vi "YKMW100 Receive String-clear buff.vi"(0 "VISA session":refnum<visa-resource-name>="MW100", 2 "Semiphore":T1, 9 "Timeout (25000)":u32=100, 11 "error in (no error)":errorcluster, 13 "Source (\"\")":string) -> (4 "dup VISA session":refnum<visa-resource-name>, 8 "Read Buffer":string, 15 "error out":errorcluster)   [LabVIEW 2009]
doc: "This VI receives ASCII code string which ends with terminator \"CRLF\" from the instrument. \nThis VI returns read buffer except CRLF."
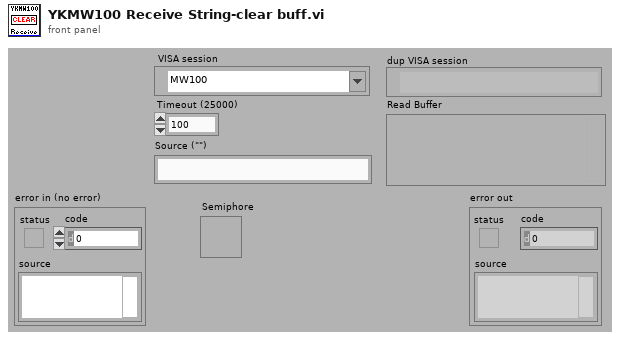
[diagram p1: front panel]
types:
  T1 = typedef "Semaphore RefNum" = refnum<k1>
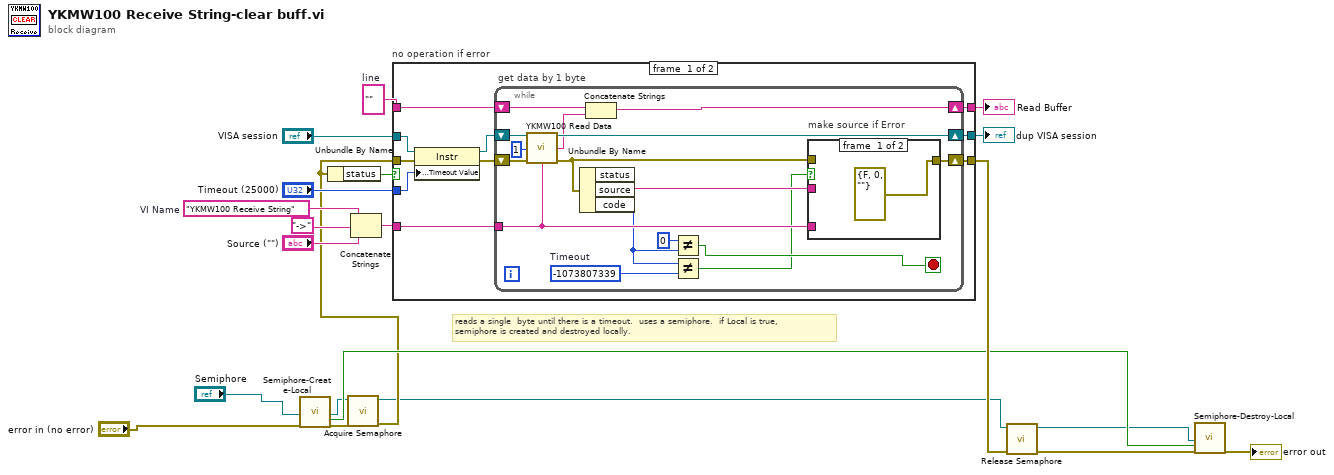
[diagram p0: block diagram]
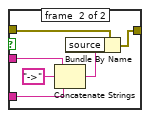
[diagram p2: hidden frame]
diagram:
  w14 = "YKMW100 Receive String"  # VI Name
  w17 = ""  # line
  # "reads a single  byte until there is a timeout.  uses a semiphore.  if Local is true, \nsemiphore is created and destroyed locally."
  n1 = call "Semiphore-Create-Local.vi"("Semiphore"="Semiphore", "error in (no error)"="error in (no error)") -> ("semaphore"=w4:T1, "Local?"=w7:bool, "error out"=w6:errorcluster)  [unwired: 15 in]
  n2 = call <vilib>:"Acquire Semaphore.vi"("error in (no error)"=w6, "semaphore"=w4) -> ("error out"=w5:errorcluster, "semaphore out"=w1:T1)  [unwired: 3 in, 1 out]
  n3 = Unbundle By Name(w5) -> ("status"=w20:bool)
  n4 = Concatenate Strings(w14, "->", "Source (\"\")") -> (w12:string)
  n5 = case "no operation if error" shown="False" w20 {
    tunnel: "VISA session" -> [w24 w57]
    tunnel: [w31 w57] -> w18
    tunnel: [w27 w56] -> w9
    tunnel: w5 -> [w26 w56]
    tunnel: w12 -> [w29 _]
    tunnel: [w28 w55] -> w19
    tunnel: w17 -> [w30 w55]
    tunnel: "Timeout (25000)" -> [w22 _]
    frame #0 {
      n6 = property class="Instr"(reference=w24, error in=w26, "General Settings:Timeout Value"=w22) -> (reference out=w23:refnum<visa-resource-name>, error out=w25:errorcluster)
      n7 = while "get data by 1 byte" {
        shift-left: w25 -> [w43]
        shift-right: [w45] -> w27
        tunnel: w29 -> [w39]
        shift-left: w30 -> [w47]
        shift-right: [w37] -> w28
        shift-right: [w42] -> w31
        shift-left: w23 -> [w44]
        stop <- w33 stop-if-true
        w36 = -1073807339  # Timeout
        n8 = call "YKMW100 Read Data.vi"("VISA session"=w44, "Byte (0)"=1, "error in (no error)"=w43, "Source (\"\")"=w39) -> ("dup VISA session"=w42:refnum<visa-resource-name>, "Read Buffer"=w38:string, "error out"=w41:errorcluster)  [unwired: 9 in]
        n9 = Unbundle By Name(w41) -> ("source"=w46:string, "code"=w35:i32)  [unwired: 1 out]
        n10 = Concatenate Strings(w47, w38) -> (w37:string)
        n11 = Not Equal?(x=0, y=w35) -> (x != y?=w33:bool)
        n12 = Not Equal?(x=w35, y=w36) -> (x != y?=w32:bool)
        n13 = case "make source if Error" shown="True" w32 {
          tunnel: w41 -> [_ w54]
          tunnel: [errorcluster {"status"=FALSE, "code"=0, "source"=""} ("error out") w53] -> w45
          tunnel: w46 -> [_ w51]
          tunnel: w39 -> [_ w49]
          frame #0 {
          }
          frame #1 {
            n14 = Concatenate Strings(w51, "->", w49) -> (w50:string)
            n15 = Bundle By Name(cluster=w54, "source"=w50) -> (w53:errorcluster)
          }
        }
      }
    }
    frame #1 {
    }
  }
  "dup VISA session" <- w18
  "Read Buffer" <- w19
  n16 = call <vilib>:"Release Semaphore.vi"("error in (no error)"=w9, "semaphore"=w1) -> ("error out"=w3:errorcluster, "semaphore out"=w2:T1)  [unwired: 4 in]
  n17 = call "Semiphore-Destroy-Local.vi"("Semiphore"=w2, "Local?"=w7, "error in (no error)"=w3) -> ("error out"=→"error out":errorcluster)  [unwired: 16 in]
